vi "Wen_main.vi"() -> ()   [LabVIEW 2024]
uses:
  <vilib>/Utility/file.llb/Read Delimited Spreadsheet (DBL).vi
  <vilib>/Utility/file.llb/Write Delimited Spreadsheet (DBL).vi
panel:
  out "x[k]时间误差波形显示":dbl[](graph)
  out "TDMS error out":errorcluster caption="错误输出"
  in  "TDMS保存路径":path
  out "回放Allan偏差曲线":cluster{"all rows":dbl[], "all rows":dbl[]}(graph)
  out "Allan偏差XY曲线显示":cluster{dbl[], dbl[]}(graph)
  in  "Allan结果CSV保存路径)":path=path "D:/EG_FPGA_Project/Project/Labview_Output/allan_result_labview.csv" caption="Allan结果CSV保存路径"
  out "error out":errorcluster caption="错误输出"
  out "二阶差分平方和sum2":dbl[](array[numeric])
  out "有效项数数组count":dbl[](array[numeric])
  out "Allan方差数组avar":dbl[](array[numeric])
  in  "数据回放":bool
  in  "计算点数上限":i32=1000000
  in  "tau0_采样间隔(s)":dbl=0.01
  out "样本数N":dbl
  in  "列索引":i32=3
  in  "csv文件路径":path=path "D:/EG_FPGA_Project/Project/下位机模拟输出/优化tdc后/ocxo_sim_time_error_tdc_measured.csv"
  out "m数组_自动读取":i32[](array[numeric])
  in  "m数组CSV路径":path=path "D:/EG_FPGA_Project/Project/Labivew_Allan/m_array_log.csv"
  out "Allan偏差数组adev":dbl[](array[numeric])
  out "tau数组":dbl[](array[numeric])
  out "二阶差分平方和sum2":dbl
  out "Allan方差avar":dbl
  out "Allan偏差adev":dbl
  out "有效项数count":dbl
  out "Allan错误信息":string
  out "tau_观测时间(s)":dbl
  out "状态编号":dbl
  out "运算完成":bool
  out "当前状态":string
  in  "紧急停止":bool
  in  "开始计算":bool
  in  "保存CSV路径":path=path "C:/Users/Administrator/Desktop/allan_result.csv"
  out "保存状态":string
  in  "结果保存":bool
  # "调试区"
  # "状\n态\n显\n示"
  # "结\n果\n显\n示"
  # "调试显示"
  # "LabView频率稳定度测量系统"
  # "参数设置"
  # "路径选择"
  # "22光电 但佳玥"
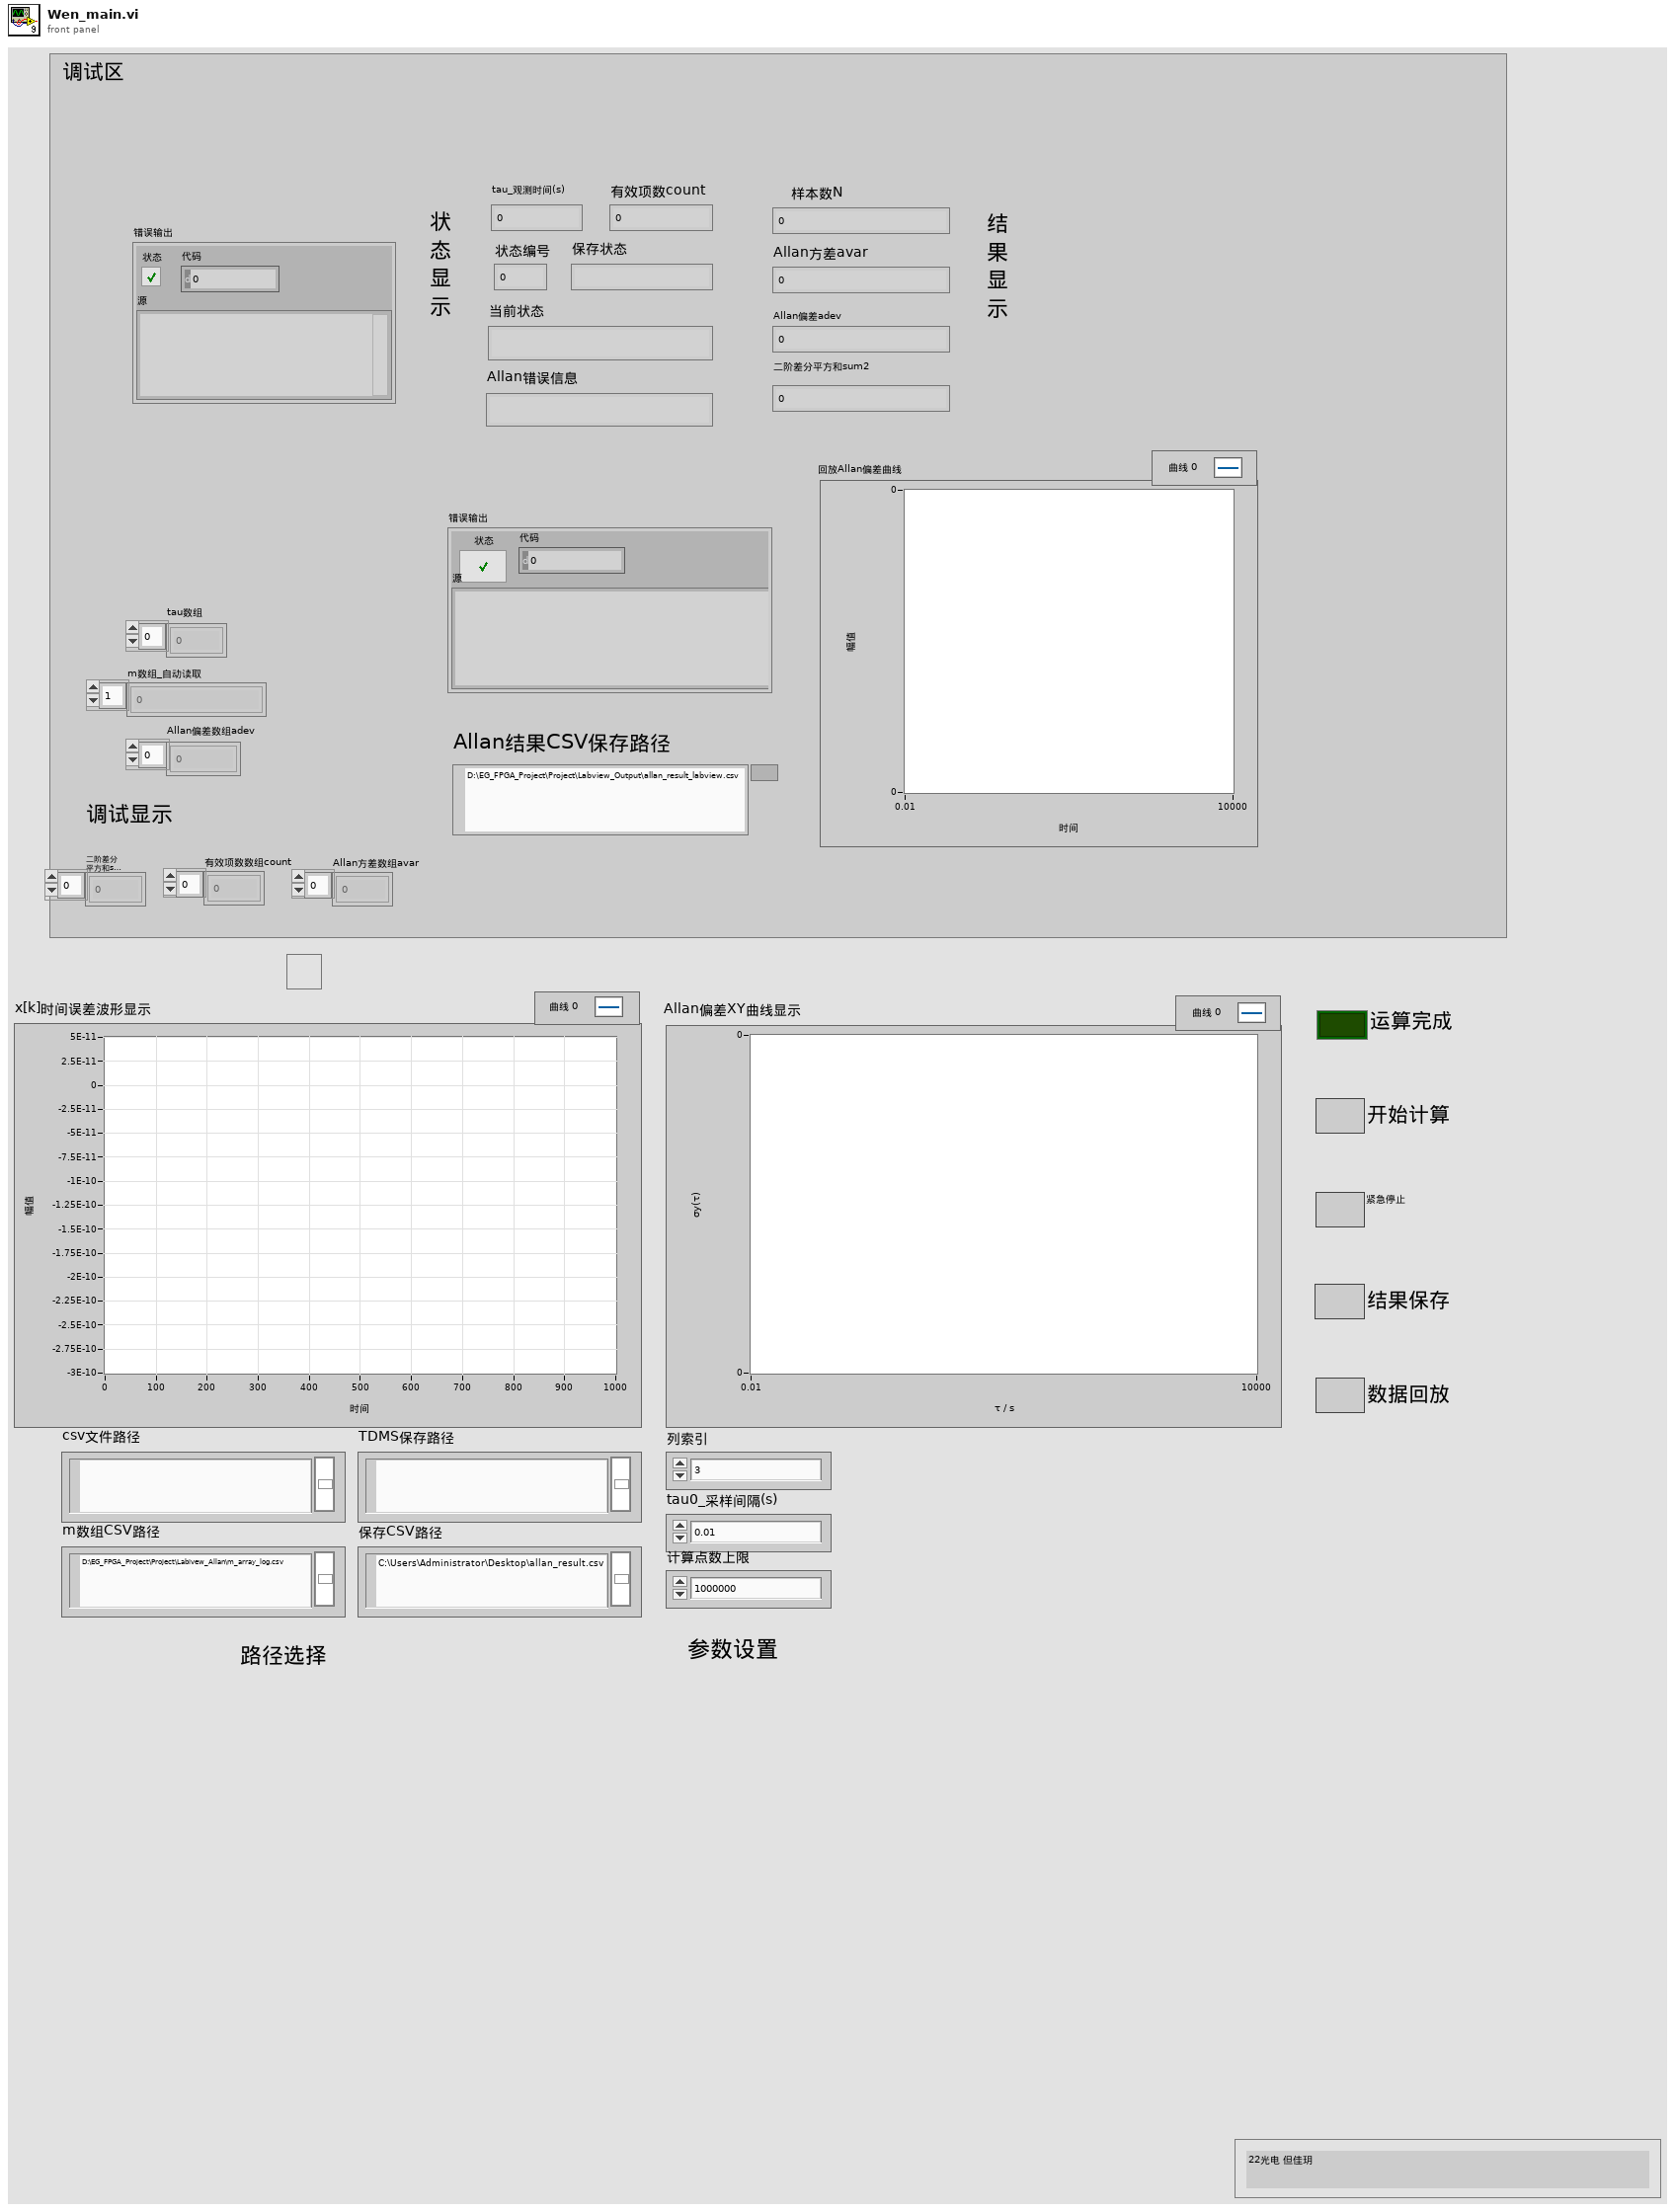
[diagram p1: front panel]
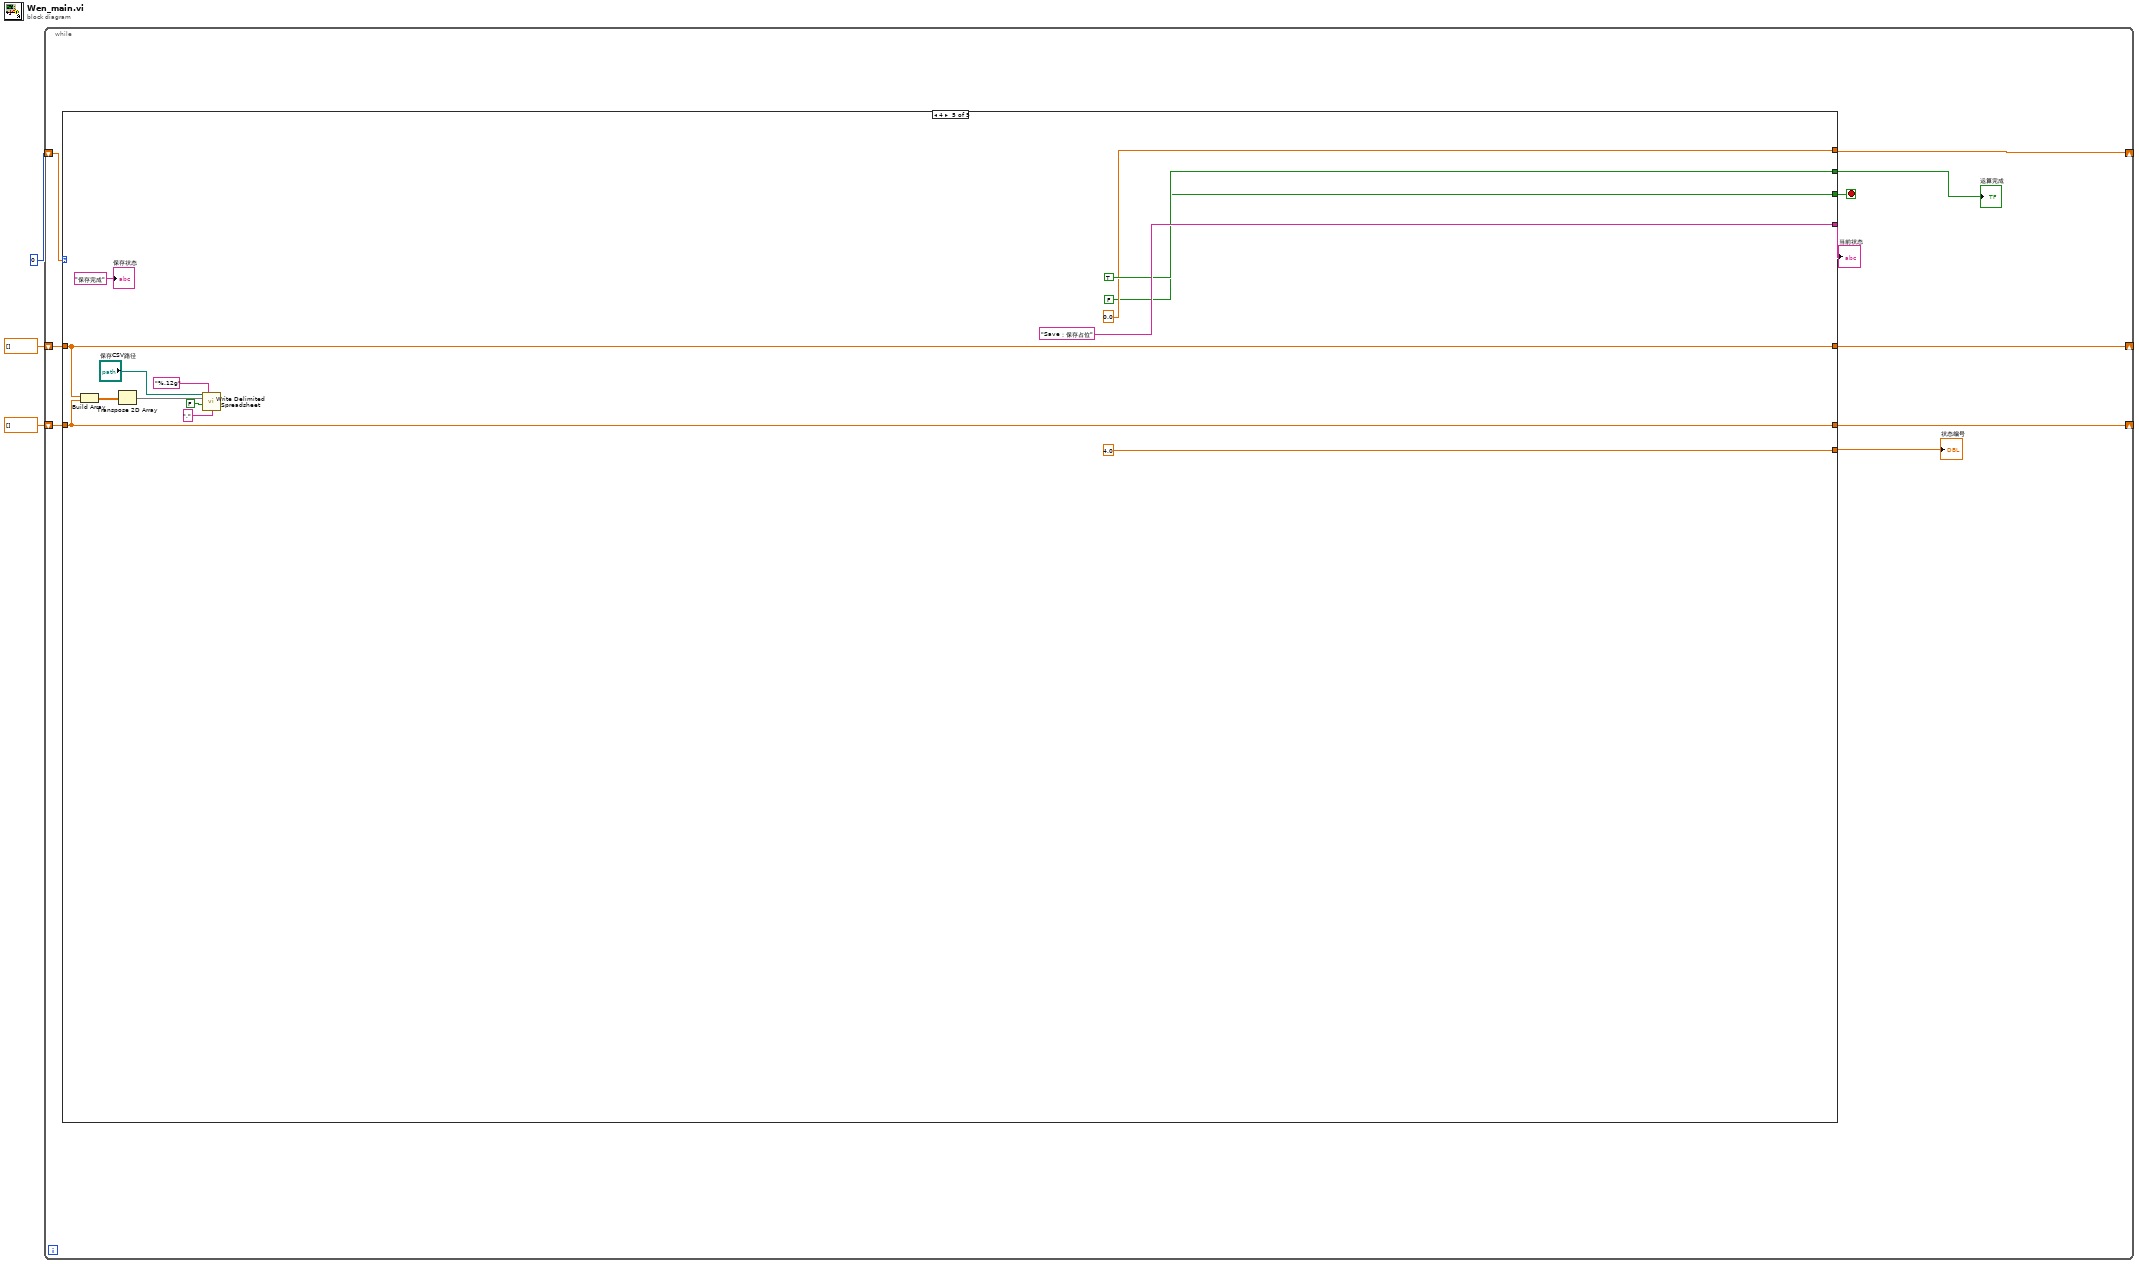
[diagram p0: block diagram]
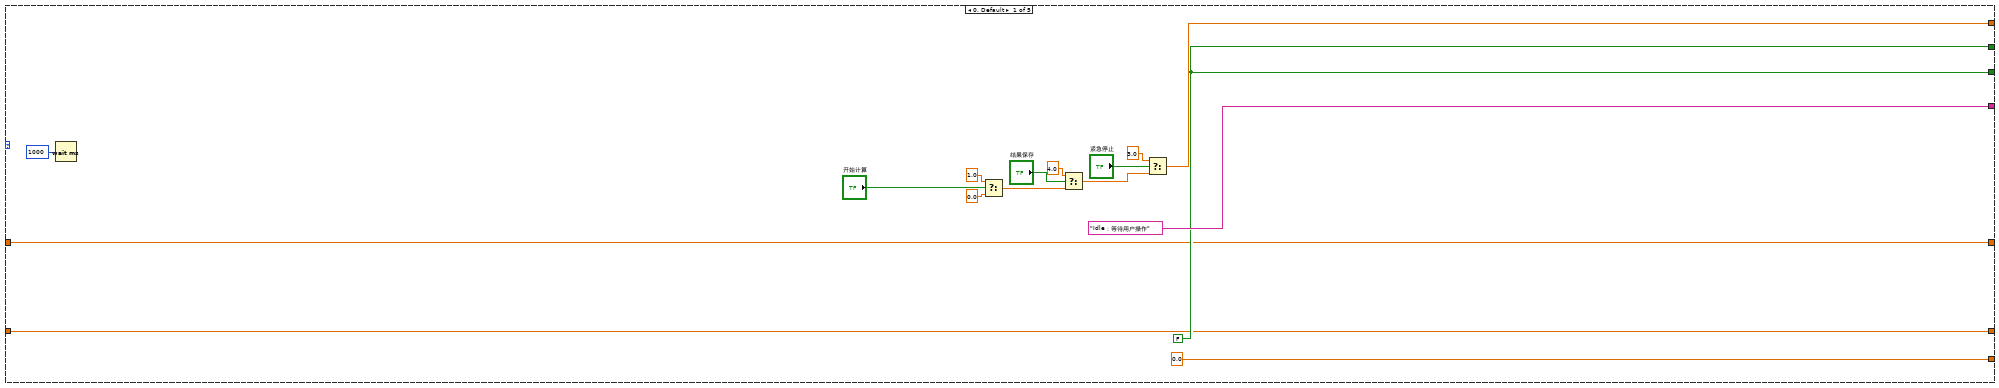
[diagram p2: hidden frame]
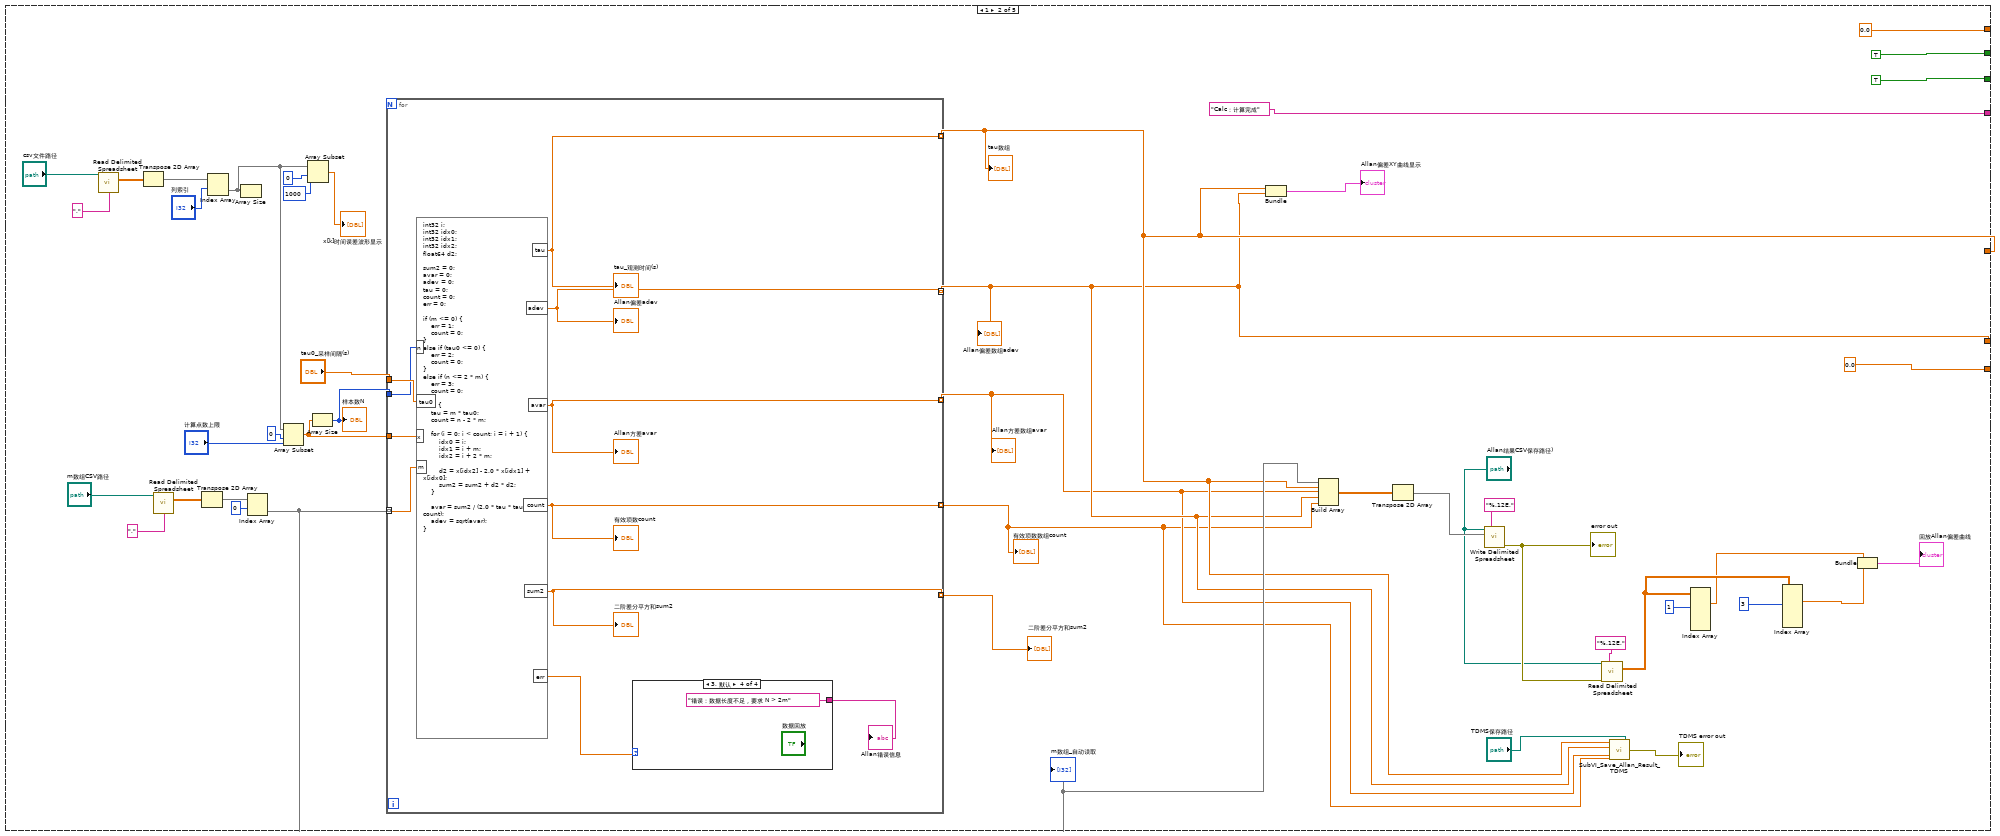
[diagram p3: hidden frame]
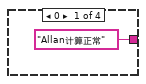
[diagram p4: hidden frame]
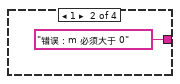
[diagram p5: hidden frame]
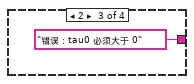
[diagram p6: hidden frame]
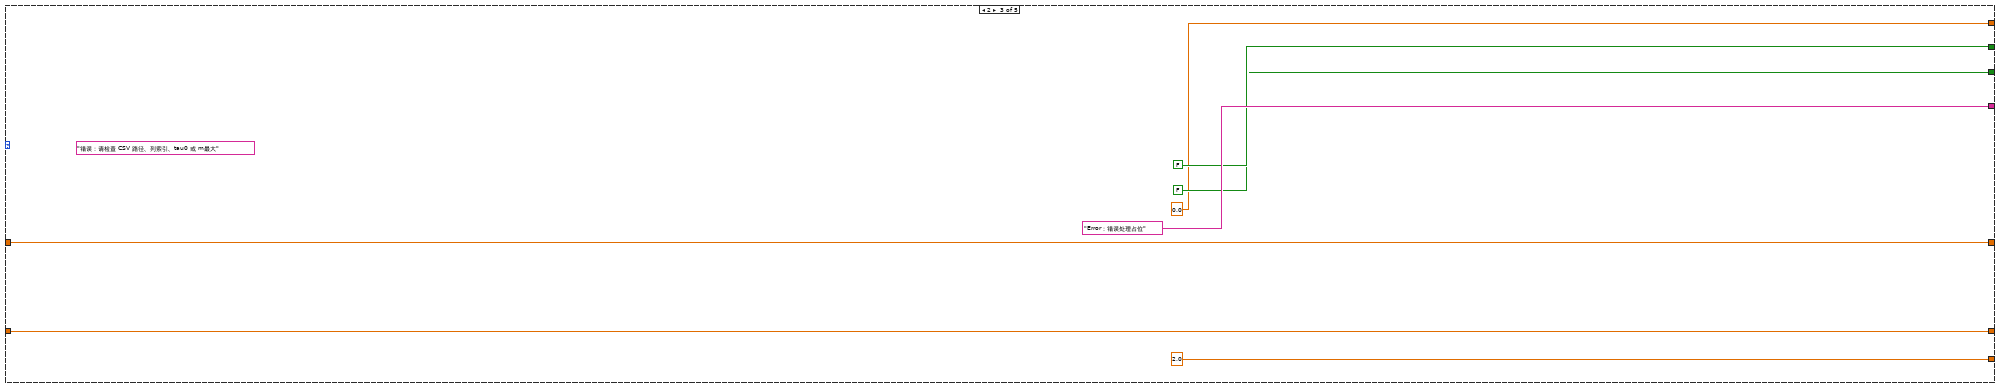
[diagram p7: hidden frame]
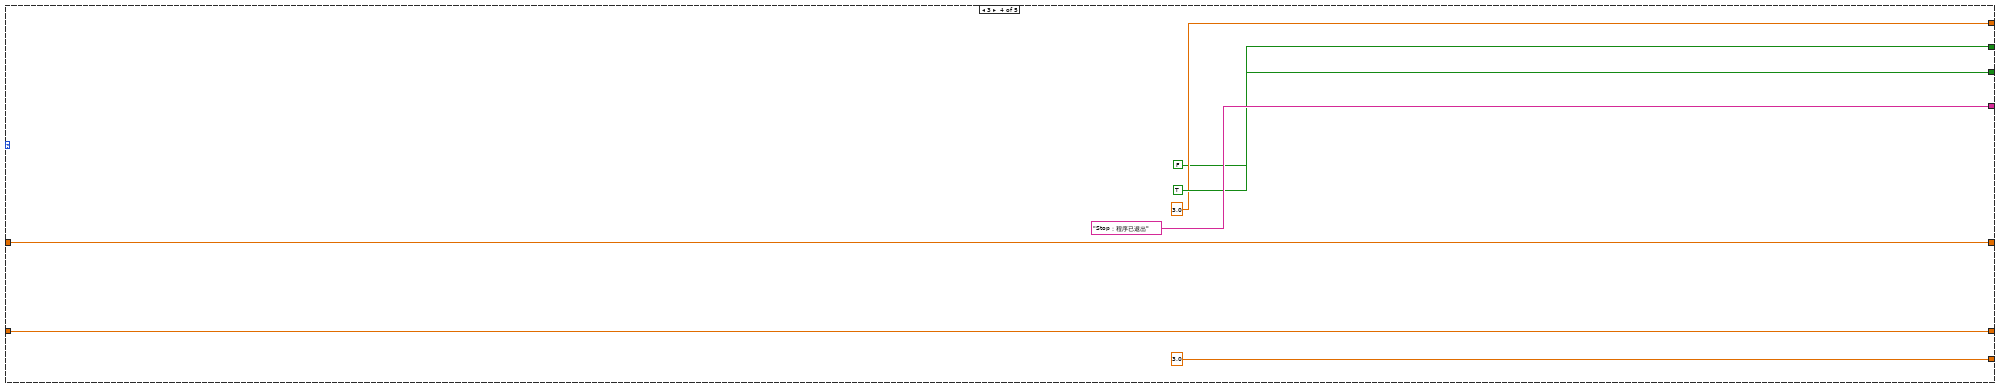
[diagram p8: hidden frame]
diagram:
  n1 = while {
    shift-right: [w4] -> _
    shift-left: 0 -> [w13]
    shift-right: [w8] -> _
    shift-left: dbl[] [] -> [w7]
    shift-right: [w6] -> _
    shift-left: dbl[] [] -> [w5]
    stop <- w10 stop-if-true
    n2 = case shown="4" w13 {
      tunnel: [w23 0.0 ("f") 0.0 ("f") 3.0 ("f") 0.0 ("f")] -> w4
      tunnel: [w17 TRUE FALSE TRUE FALSE] -> w10
      tunnel: ["Idle：等待用户操作" "Calc：计算完成" "Error：错误处理占位" "Stop：程序已退出" "Save：保存占位"] -> w12
      tunnel: [0.0 ("状态编号") 0.0 ("状态编号") 2.0 ("状态编号") 3.0 ("状态编号") 4.0 ("状态编号")] -> w11
      tunnel: [w17 TRUE FALSE FALSE TRUE] -> w9
      tunnel: [w16 w35 w91 w98 w107] -> w8
      tunnel: w7 -> [w16 _ w91 w98 w107]
      tunnel: [w15 w34 w90 w97 w106] -> w6
      tunnel: w5 -> [w15 _ w90 w97 w106]
      frame 0, Default {
        w17 = FALSE
        n3 = Wait (ms)(milliseconds to wait=u32 1000 ("等待时间（毫秒）")) -> ()  [unwired: 1 out]
        n4 = Select(t=1.0, s="开始计算", f=0.0) -> (s? t:f=w24:dbl)
        n5 = Select(t=4.0, s="结果保存", f=w24) -> (s? t:f=w21:dbl)
        n6 = Select(t=3.0, s="紧急停止", f=w21) -> (s? t:f=w23:dbl)
      }
      frame 1 {
        n7 = call-poly <vilib>:"Read Delimited Spreadsheet.vi"("file path (dialog if empty)"="csv文件路径", "delimiter (\\t)"="," ("delimiter (\\t)")) -> ("all rows"=w64:dbl[][])  [unwired: 8 in, 5 out]
        n8 = Transpose 2D Array(2D array=w64) -> (transposed array=w61:dbl[][])
        n9 = call-poly <vilib>:"Read Delimited Spreadsheet.vi"("file path (dialog if empty)"="m数组CSV路径", "delimiter (\\t)"="," ("delimiter (\\t)")) -> ("all rows"=w68:dbl[][])  [unwired: 8 in, 5 out]
        n10 = Transpose 2D Array(2D array=w68) -> (transposed array=w66:dbl[][])
        n11 = Index Array(array=w61, index (row)="列索引") -> (element=w57:dbl[])  [unwired: 1 in]
        n12 = Array Size(array=w57) -> ()  [unwired: 1 out]
        n13 = Index Array(array=w66, index (row)=0 ("索引")) -> (element=w50:dbl[])  [unwired: 1 in]
        "m数组_自动读取" <- w50
        n14 = Array Subset(array=w57, index=0 ("索引"), length="计算点数上限") -> (w52:dbl[])
        n15 = Array Subset(array=w57, index=0 ("索引"), length=1000 ("长度")) -> (→"x[k]时间误差波形显示":dbl[])
        n16 = Array Size(array=w52) -> (size(s)=w53:i32)
        "样本数N" <- w53
        n17 = for {
          tunnel: [w83] -> w35 mode=indexing
          tunnel: [w82] -> w34 mode=indexing
          tunnel: "tau0_采样间隔(s)" -> [w81]
          tunnel: w53 -> [w78]
          tunnel: w52 -> [w80]
          tunnel: w50 -> [w79] mode=indexing
          tunnel: [w77] -> w33 mode=indexing
          tunnel: [w76] -> w32 mode=indexing
          tunnel: [w75] -> w51 mode=indexing
          n18 = formula code="int32 i;\nint32 idx0;\nint32 idx1;\nint32 idx2;\nfloat64 d2;\n\nsum2 = 0;\navar = 0;\nadev = 0;\ntau = 0;\ncount = 0;\nerr = 0;\n\nif (m <= 0) {\n    err = 1;\n    count = 0;\n}\nelse if (tau0 <= 0) {\n    err = 2;\n    count = 0;\n}\nelse if (n <= 2 * m) {\n    err = 3;\n    count = 0;\n}\nelse {\n    tau = m * tau0;\n    count = n - 2 * m;\n\n    for (i = 0; i < count; i = i + 1) {\n        idx0 = i;\n        idx1 = i + m;\n        idx2 = i + 2 * m;\n\n        d2 = x[idx2] - 2.0 * x[idx1] + x[idx0];\n        sum2 = sum2 + d2 * d2;\n    }\n\n    avar = sum2 / (2.0 * tau * tau * count);\n    adev = sqrt(avar);\n}"("x"=w80, "tau0"=w81, "m"=w79, "n"=w78) -> ("tau"=w83:dbl, "avar"=w77:dbl, "adev"=w82:dbl, "count"=w76:dbl, "sum2"=w75:dbl, "err"=w84:dbl)
          "二阶差分平方和sum2" <- w75
          "Allan方差avar" <- w77
          "Allan偏差adev" <- w82
          "有效项数count" <- w76
          "tau_观测时间(s)" <- w83
          n19 = case shown="3, 默认" w84 {
            tunnel: ["Allan计算正常" "错误：m 必须大于 0" "错误：tau0 必须大于 0" "错误：数据长度不足，要求 N > 2m"] -> w85
            frame 0 {
            }
            frame 1 {
            }
            frame 2 {
            }
            frame 3, Default {
            }
          }
          "Allan错误信息" <- w85
        }
        "tau数组" <- w35
        "Allan偏差数组adev" <- w34
        "Allan方差数组avar" <- w33
        "有效项数数组count" <- w32
        "二阶差分平方和sum2" <- w51
        n20 = Bundle(w35, w34) -> (→"Allan偏差XY曲线显示":cluster{dbl[], dbl[]})  [unwired: 1 in]
        n21 = Build Array(w50, w35, w33, w34, w32) -> (w49:dbl[][])
        n22 = Transpose 2D Array(2D array=w49) -> (transposed array=w48:dbl[][])
        n23 = call-poly <vilib>:"Write Delimited Spreadsheet.vi"("file path (dialog if empty)"="Allan结果CSV保存路径)", "format (%.3f)"="%.12E,", "2D data"=w48) -> ("error out"=w45:errorcluster)  [unwired: 11 in, 1 out]
        "error out" <- w45
        n24 = call-poly <vilib>:"Read Delimited Spreadsheet.vi"("file path (dialog if empty)"="Allan结果CSV保存路径)", "format (%.3f)"="%.12E,", "error in (no error)"=w45) -> ("all rows"=w42:dbl[][])  [unwired: 7 in, 5 out]
        n25 = call "SubVI_Save_Allan_Result_TDMS.vi"("TDMS保存路径"="TDMS保存路径", "num_pairs"=w32, "allan_variance"=w33, "allan_deviation"=w34, "tau_s"=w35) -> ("error out"=→"TDMS error out":errorcluster)  [unwired: 1 in]
        n26 = Index Array(array=w42, index (col) #1=1 ("索引 (列)")) -> (element #1=w41:dbl[])  [unwired: 5 in, 2 out]
        n27 = Index Array(array=w42, index (col) #1=3 ("索引 (行)")) -> (element #1=w40:dbl[])  [unwired: 5 in, 2 out]
        n28 = Bundle("all rows"=w41, "all rows"=w40) -> (→"回放Allan偏差曲线":cluster{"all rows":dbl[], "all rows":dbl[]})  [unwired: 1 in]
      }
      frame 2 {
        (unwired) "错误：请检查 CSV 路径、列索引、tau0 或 m最大"
      }
      frame 3 {
      }
      frame 4 {
        n29 = Build Array(w107, w106) -> (w105:dbl[][])
        n30 = Transpose 2D Array(2D array=w105) -> (transposed array=w104:dbl[][])
        n31 = call-poly <vilib>:"Write Delimited Spreadsheet.vi"("file path (dialog if empty)"="保存CSV路径", "format (%.3f)"="%.12g", "2D data"=w104, "append to file? (new file:F)"=FALSE, "delimiter (\\t)"="," ("delimiter (\\t)")) -> ()  [unwired: 9 in, 2 out]
        "保存状态" <- "保存完成"
      }
    }
    "当前状态" <- w12
    "状态编号" <- w11
    "运算完成" <- w9
  }
